vi "PQfinish.vi"(8 "error in (no error)":errorcluster, 11 "conn":u32) -> (0 "error out":errorcluster)   [LabVIEW 2019, in "libpqlv.lvlib"]
doc: "Closes the connection to the server. Also frees memory used by the PGconn object."
uses:
  libpqlv.lvlib
  libpq.dll
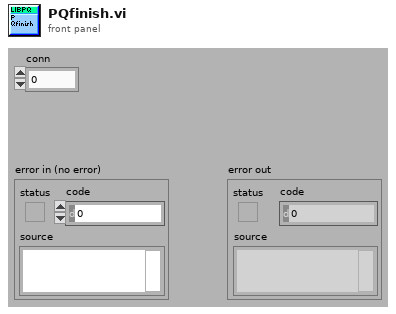
[diagram p1: front panel]
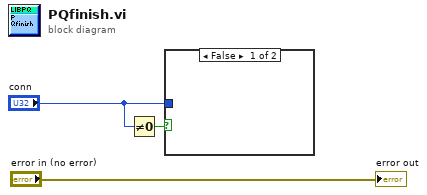
[diagram p0: block diagram]
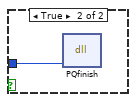
[diagram p2: hidden frame]
diagram:
  n1 = Not Equal To 0?(x="conn") -> (x != 0?=w2:bool)
  n2 = case shown="False" w2 {
    tunnel: "conn" -> [_ w4]
    frame False {
    }
    frame True {
      n3 = dll-call lib="libpq.*" fn="PQfinish"("conn"=w4) -> ()  [unwired: 5 in, 2 out]
    }
  }
  "error out" <- "error in (no error)"
